vi "parse_Bar.vi"(8 "error in":errorcluster, 11 "msg in":string) -> (0 "error out":errorcluster, 2 "Bar":T1, 3 "msg out":string)   [LabVIEW 2016]
doc: "Parses a message into a bar"
uses:
  std_msgs/subs/parse_string_scalar.vi
  std_msgs/subs/parse_i32_scalar.vi
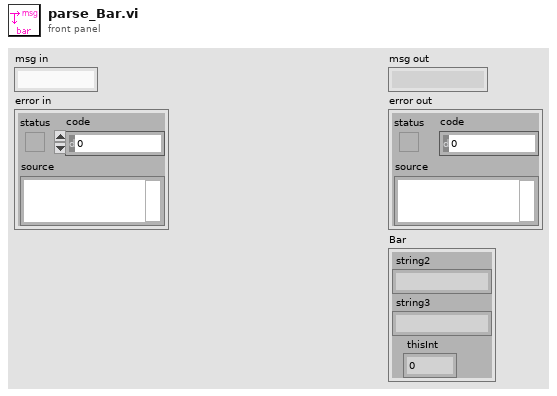
[diagram p1: front panel]
types:
  T1 = cluster{" string2":string, " string3":string, " thisInt":i32}
  T2 = cluster{"string":string, "string":string, "number":i32}
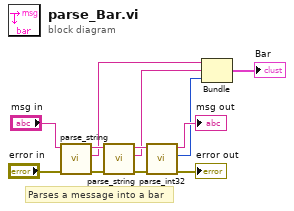
[diagram p0: block diagram]
diagram:
  # "Parses a message into a bar"
  n1 = call-poly "parse_string.vi"("error in"="error in", "msg in"="msg in") -> ("error out"=w9:errorcluster, "string"=w4:string, "msg out"=w10:string)  [unwired: 3 in]
  n2 = call-poly "parse_string.vi"("error in"=w9, "msg in"=w10) -> ("error out"=w7:errorcluster, "string"=w3:string, "msg out"=w8:string)  [unwired: 3 in]
  n3 = call-poly "parse_int32.vi"("error in"=w7, "msg in"=w8) -> ("error out"=→"error out":errorcluster, "number"=w2:i32, "msg out"=→"msg out":string)  [unwired: 3 in]
  n4 = Bundle("string"=w4, "string"=w3, "number"=w2) -> (→"Bar":T2)  [unwired: 1 in]
